vi "MoveState_test.vi"(3 "Delay [ms]":i32=30 min=0, 5 "Control unit ID":i32=1 min=1 max=10) -> (0 "Move state 3":i32, 1 "Move state 2":i32, 2 "Move state 1":i32)   [LabVIEW 2020]
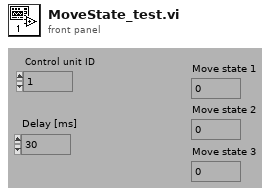
[diagram p1: front panel]
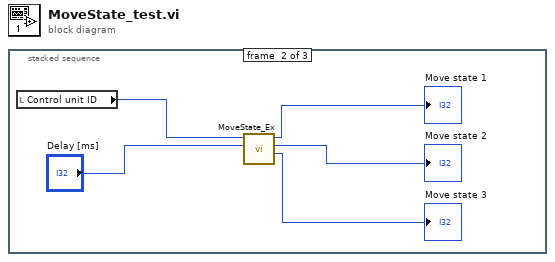
[diagram p0: block diagram]
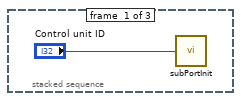
[diagram p2: hidden frame]
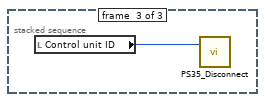
[diagram p3: hidden frame]
diagram:
  n1 = stacked-sequence {
    frame #0 {
      n2 = call "subPortInit.vi"("Control unit ID"="Control unit ID") -> ()  [unwired: 2 out]
    }
    frame #1 {
      n3 = local read "Control unit ID"() -> (w6:i32)
      n4 = call "MoveState_Ex.vi"("Delay [ms]"="Delay [ms]", "Control unit ID"=w6) -> ("Move state 3"=→"Move state 3":i32, "Move state 2"=→"Move state 2":i32, "Move state 1"=→"Move state 1":i32)  [unwired: 2 in, 1 out]
    }
    frame #2 {
      n5 = local read "Control unit ID"() -> (w7:i32)
      n6 = call "PS35_Disconnect.vi"("Control unit ID"=w7) -> ()  [unwired: 2 in, 1 out]
    }
  }
